vi "FinalCheck.vi"(8 "errin":errorcluster, 10 "L2T":T1 caption="Limites de test pris en compte", 11 "SN":string="0B5MEVA000CA1JC1M0000041") -> (0 "error out":errorcluster, 2 "intrafinal":string, 3 "ET logique":bool, 4 "données":string[](array[string]), 6 "tableau ajouté":bool[](array[boolean]))   [LabVIEW 2020]
uses:
  <vilib>/regexp/Match Regular Expression.xnode
  VarGLO/Global var.vi
  subVI/Ctrl/L2T.ctl
panel:
  # "Pre DCIR_____________________________________"
  # "intra DCIR_____________________________________"
  # "Post DCIR_____________________________________"
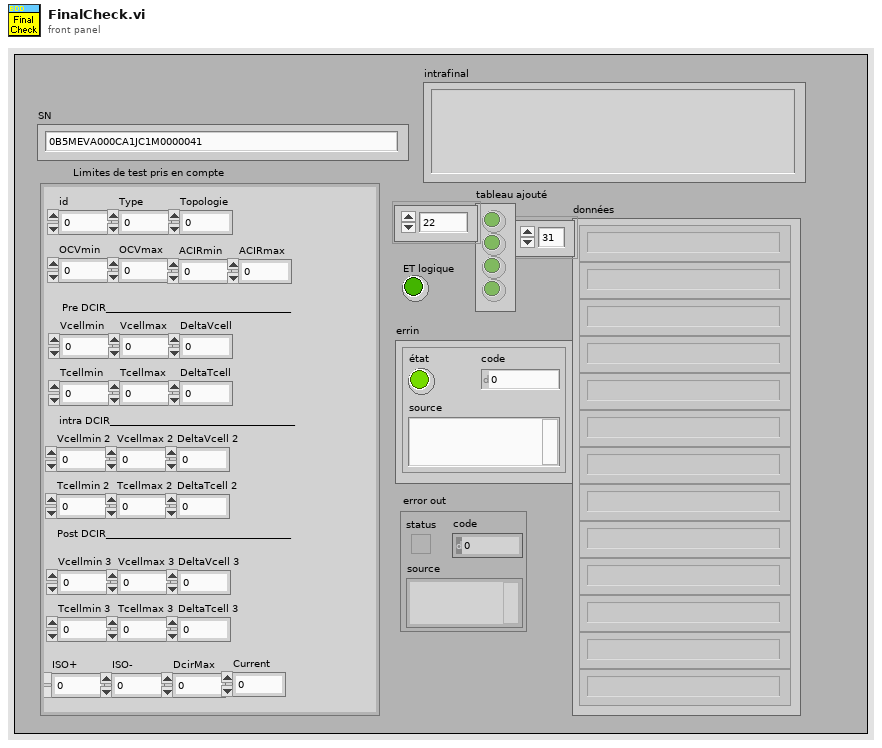
[diagram p1: front panel]
types:
  T1 = typedef "L2T.ctl" = cluster{"id":dbl, "Type":dbl, "OCVmin":dbl, "OCVmax":dbl, "ACIRmin":dbl, "ACIRmax":dbl, "Vcellmin":dbl, "Vcellmax":dbl, "DeltaVcell":dbl, "Tcellmin":dbl, "Tcellmax":dbl, "DeltaTcell":dbl, "ISO+":dbl, "ISO-":dbl, "DcirMax":dbl, "Current":dbl, "Topologie":dbl, "Vcellmin 2":dbl, "Vcellmax 2":dbl, "DeltaVcell 2":dbl, "Tcellmin 2":dbl, "Tcellmax 2":dbl, "DeltaTcell 2":dbl, "Vcellmin 3":dbl, "Vcellmax 3":dbl, "DeltaVcell 3":dbl, "Tcellmin 3":dbl, "Tcellmax 3":dbl, "DeltaTcell 3":dbl}
  T2 = cluster{"[0]":dbl, "[1]":dbl, "[2]":dbl, "[3]":dbl, "[4]":dbl, "[5]":dbl, "[6]":dbl, "[7]":dbl, "[8]":dbl, "[9]":dbl, "[10]":dbl, "[11]":dbl, "[12]":dbl, "[13]":dbl, "[14]":dbl, "[15]":dbl, "[16]":dbl, "[17]":dbl, "[18]":dbl, "[19]":dbl, "[20]":dbl, "[21]":dbl, "[22]":dbl, "[23]":dbl}
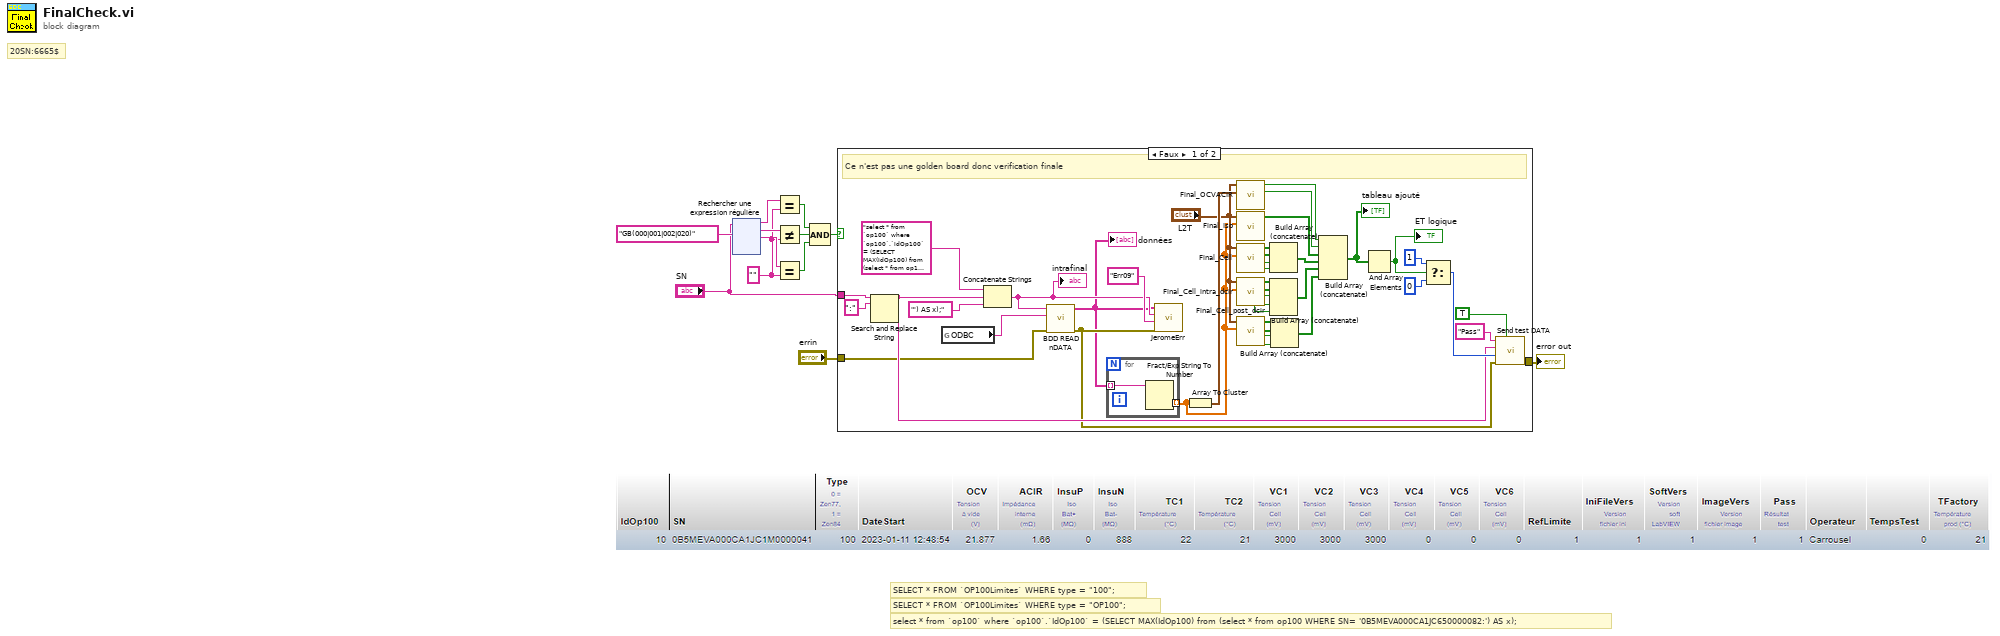
[diagram p0: block diagram]
diagram:
  w8 = "" ("y")
  # "select * from `op100` where `op100`.`IdOp100` = (SELECT MAX(IdOp100) from (select * from op100 WHERE SN= '0B5MEVA000CA1JC650000082:') AS x);"
  # "SELECT * FROM `OP100Limites` WHERE type = \"OP100\";"
  # "SELECT * FROM `OP100Limites` WHERE type = \"100\";"
  # "20SN:6665$"
  n1 = xnode "Rechercher une expression régulière"("chaîne en entrée"="SN", "expression régulière"="GB(000|001|002|020)") -> ("avant la correspondance"=w7:string, "toute l'expression"=w9:string, "après la correspondance"=w10:string)  [unwired: 4 in, 2 out]
  n2 = Equal? ("Égaux ?")(x=w7, y=w8) -> (x = y?=w6:bool)
  n3 = Not Equal?(x=w9, y=w8) -> (x != y?=w5:bool)
  n4 = Equal? ("Égaux ?")(x=w10, y=w8) -> (x = y?=w4:bool)
  n5 = Compound Arithmetic op=AND ("Opérateur arithmétique")(w6, w5, w4) -> (w3:bool)
  n6 = case shown="Faux" w3 {
    tunnel: [w39 w56] -> w12
    tunnel: "errin" -> [w36 w56]
    tunnel: "SN" -> [w37 _]
    frame False {
      # "Ce n'est pas une golden board donc verification finale"
      n7 = Search and Replace String ("Rechercher et remplacer une chaîne")(input string=w37, search string=":" ("chaîne recherchée")) -> (result string=w40:string)  [unwired: 6 in, 3 out]
      n8 = global read "Global var.vi" "ODBC"() -> (w13:string)
      n9 = Concatenate Strings("select * from `op100` where `op100`.`IdOp100` = (SELECT MAX(IdOp100) from (select * from op100 WHERE SN= '" ("SQL query"), w40, "') AS x);" ("chaîne")) -> (w35:string)
      "intrafinal" <- w35
      n10 = call <userlib>:"BDD READ nDATA.vi"("errin"=w36, "DSN name"=w13, "Instruction"=w35) -> ("error out"=w34:errorcluster, "Array"=w14:string[])  [unwired: 7 in]
      "données" <- w14
      n11 = for {
        tunnel: w14 -> [w55] mode=indexing
        tunnel: [w54] -> w16 mode=indexing
        n12 = Fract/Exp String To Number(string=w55) -> (number=w54:dbl)  [unwired: 3 in, 1 out]
      }
      n13 = call "JeromeErr.vi"("Errin"=w34, "CodeERR"="Err09", "RequetteSQL"=w35, "RetourSQL"=w14) -> ()  [unwired: 8 in]
      n14 = Array To Cluster ("Tableau en cluster")(array=w16) -> (cluster=w33:T2)
      n15 = call "Final_OCVACIR.vi"("Cluster"=w33, "L2T"="L2T") -> ("Boolean"=w49:bool, "Boolean 2"=w50:bool)  [unwired: 8 in]
      n16 = call "Final_Iso.vi"("Array in"=w16, "L2T"="L2T") -> ("Array out"=w48:bool[])  [unwired: 9 in]
      n17 = call "Final_Cell.vi"("Array in"=w16, "L2T"="L2T") -> ("DeltaTcell"=w20:bool, "DeltaVcell"=w21:bool, "Vcell"=w22:bool[], "Tcell"=w23:bool[])  [unwired: 6 in]
      n18 = call "Final_Cell_intra_dcir.vi"("Array in"=w16, "L2T"="L2T") -> ("DeltaTcell"=w27:bool, "DeltaVcell"=w26:bool, "Vcell"=w25:bool[], "Tcell"=w24:bool[], "Dcir"=w15:bool)  [unwired: 5 in]
      n19 = call "Final_Cell_post_dcir.vi"("Array in"=w16, "L2T"="L2T") -> ("DeltaTcell"=w31:bool, "DeltaVcell"=w30:bool, "Vcell"=w29:bool[], "Tcell"=w28:bool[])  [unwired: 6 in]
      n20 = Build Array (concatenate)(w23, w22, w21, w20) -> (w19:bool[])
      n21 = Build Array (concatenate)(w24, w25, w26, w27, w15) -> (w18:bool[])
      n22 = Build Array (concatenate)(w28, w29, w30, w31) -> (w17:bool[])
      n23 = Build Array (concatenate)(w50, w49, w48, w19, w18, w17) -> (w51:bool[])
      "tableau ajouté" <- w51
      n24 = And Array Elements ("ET logique entre les éléments du tableau")(Boolean array=w51) -> (logical AND=w46:bool)
      "ET logique" <- w46
      n25 = Select ("Sélectionner")(t=u8 1 ("cas vrai"), s=w46, f=u8 0 ("cas faux")) -> (s? t:f=w43:u8)
      n26 = call "Send test DATA.vi"("isInt?"=TRUE, "errin"=w34, "Value"=w43, "SN"=w40, "test"="Pass") -> ("error out"=w39:errorcluster)  [unwired: 6 in]
    }
    frame True {
      # "On fait pas de verif finale car Golden Board"
    }
  }
  "error out" <- w12
